vi "Funkcja blocking nie dziala.vi"() -> ()   [LabVIEW 2009, in "MicroDAQ.lvlib"]
uses:
  <instrlib>/MicroDAQ/MicroDAQ.lvlib
  <instrlib>/MicroDAQ/Tools/Analo Range Enum.ctl
  <instrlib>/MicroDAQ/MLink32.dll
  <instrlib>/MicroDAQ/Mlink library wraper/mlink.lvlib
panel:
  out "Czas wykonywania sie write [ms]":u32
  out "error out":errorcluster
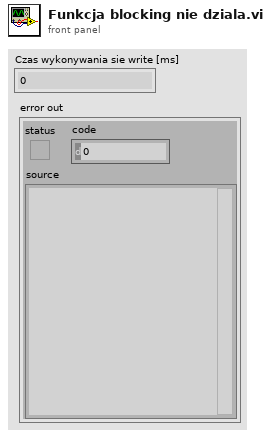
[diagram p1: front panel]
types:
  T1 = typedef "MicroDAQ.lvlib/Analo Range Enum.ctl" = enum16{"±10V", "0-10V", "±5V", "0-5V", "±5.12V", "±2.56V", "±2.5V", "±2V", "±1.24V", "±0.64V"}
  T2 = enum16{"non-blocking / no index reset", "blocking / index reset"}
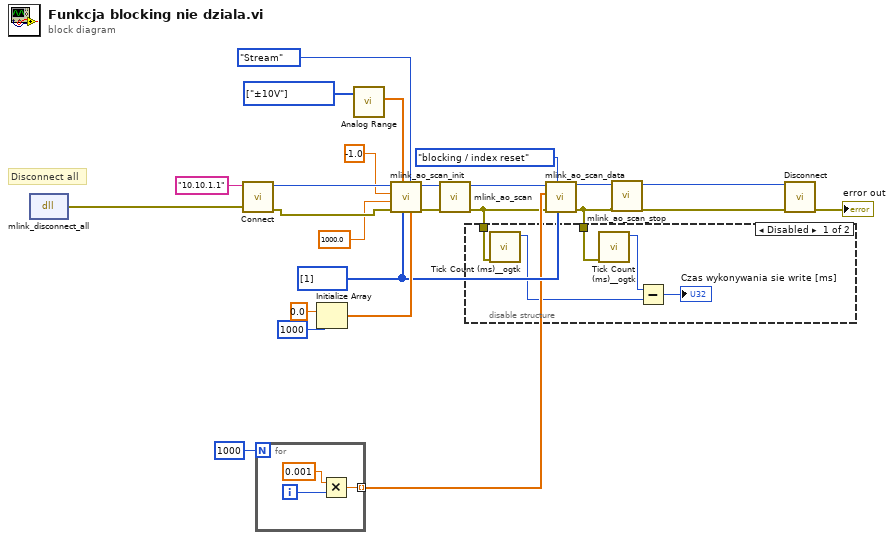
[diagram p0: block diagram]
diagram:
  w8 = u8[] [1] ("channels")
  w15 = T1[] [enum."±10V"] items=["±10V", "0-10V", "±5V", "0-5V", "±5.12V", "±2.56V", "±2.5V", "±2V", "±1.24V", "±0.64V"] ("ranges in")
  # "Disconnect all"
  n1 = dll-call lib="C:/Program Files (x86)/National Instruments/LabVIEW 2009/instr.lib/MicroDAQ/MLink32.dll" fn="mlink_disconnect_all" ("MLink32.*:mlink_connect")() -> (error out=w23:errorcluster)  [unwired: 4 in, 1 out]
  n2 = call <instrlib>:"Connect.vi"("error in (no error)"=w23, "IP address"="10.10.1.1") -> ("error out"=w21:errorcluster, "connection ID"=w22:i32)  [unwired: 8 in]
  n3 = for {
    N: 1000 ("dimension size") -> [_]
    tunnel: [w26] -> w6 mode=indexing
    i -> [w28]
    n4 = Multiply(x=0.001 ("element"), y=w28) -> (x*y=w26:dbl)
  }
  n5 = Initialize Array(0.0 ("element"), 1000 ("dimension size")) -> (w11:dbl[])
  n6 = call <instrlib>:"Analog Range.vi"("ranges in"=w15) -> ("range Array out"=w14:dbl[])  [unwired: 10 in]
  n7 = call <instrlib>:"mlink_ao_scan_init.vi"("data"=w11, "mode"=enum16{"Periodic", "Stream"}."Stream", "channels"=w8, "range"=w14, "error in (no error)"=w21, "rate"=1000.0, "duration"=-1.0, "connection ID"=w22) -> ("error out"=w19:errorcluster, "connection ID out"=w20:i32)  [unwired: 2 in]
  n8 = call <instrlib>:"mlink_ao_scan.vi"("error in (no error)"=w19, "connection ID"=w20) -> ("error out"=w5:errorcluster, "connection ID out"=w9:i32)  [unwired: 8 in]
  n9 = call <instrlib>:"mlink_ao_scan_data.vi"("channels"=w8, "opt"=T2."blocking / index reset", "error in (no error)"=w5, "data"=w6, "connection ID"=w9) -> ("error out"=w4:errorcluster, "connection ID out"=w3:i32)  [unwired: 5 in]
  n10 = disable-structure shown="Disabled" {
    disable-tunnel: w5 -> [w33 _]
    disable-tunnel: w4 -> [w29 _]
    frame #0 {
      n11 = call <userlib>:"Tick Count (ms)__ogtk.vi"("error in (no error)"=w33) -> ("millisecond timer value"=w31:u32)  [unwired: 9 in, 1 out]
      n12 = call <userlib>:"Tick Count (ms)__ogtk.vi"("error in (no error)"=w29) -> ("millisecond timer value"=w32:u32)  [unwired: 9 in, 1 out]
      n13 = Subtract(x=w32, y=w31) -> (x-y=→"Czas wykonywania sie write [ms]":u32)
    }
    frame #1 {
    }
  }
  n14 = call <instrlib>:"mlink_ao_scan_stop.vi"("error in (no error)"=w4, "connection ID"=w3) -> ("error out"=w1:errorcluster, "connection ID out"=w2:i32)  [unwired: 8 in]
  n15 = call <instrlib>:"Disconnect.vi"("error in (no error)"=w1, "connection ID"=w2) -> ("error out"=→"error out":errorcluster)  [unwired: 9 in]
